vi "7 Segment LED - Automatic Counter.vi"() -> ()   [LabVIEW 2016]
panel:
  in  "STOP":bool
  out "f":bool
  out "e":bool
  out "c":bool
  out "b":bool
  out "d":bool
  out "g":bool
  out "a":bool
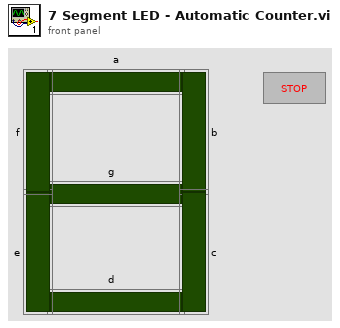
[diagram p1: front panel]
types:
  T1 = enum16{"ZERO", "ONE", "TWO", "THREE", "FOUR", "FIVE", "SIX", "SEVEN", "EIGHT", "NINE"}
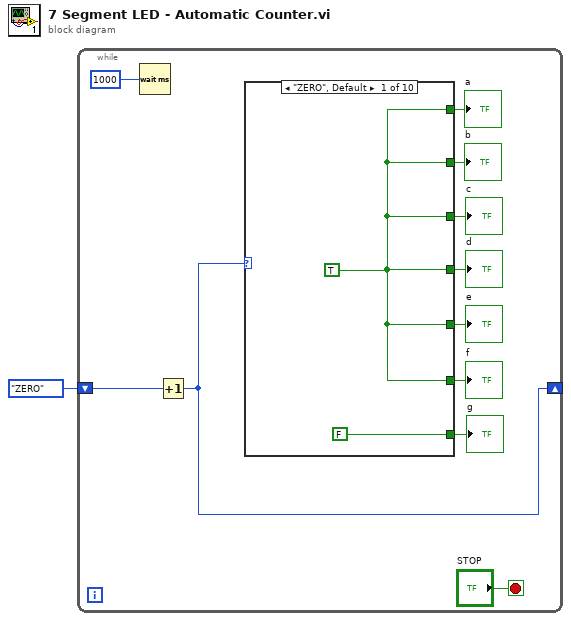
[diagram p0: block diagram]
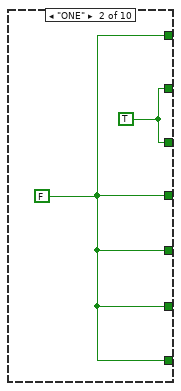
[diagram p2: hidden frame]
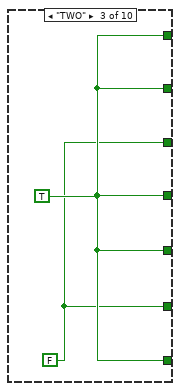
[diagram p3: hidden frame]
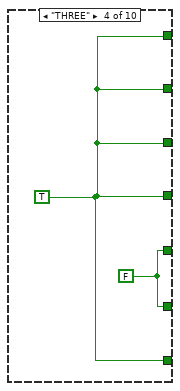
[diagram p4: hidden frame]
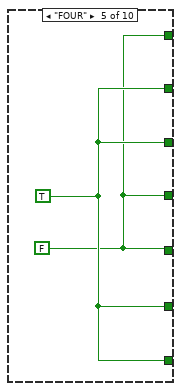
[diagram p5: hidden frame]
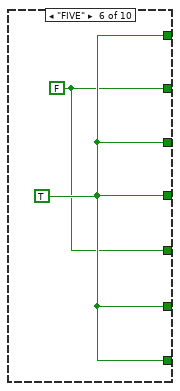
[diagram p6: hidden frame]
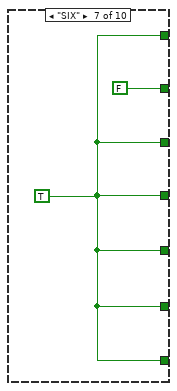
[diagram p7: hidden frame]
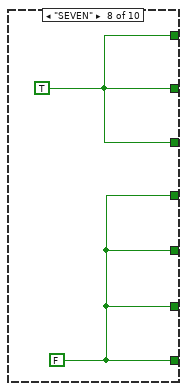
[diagram p8: hidden frame]
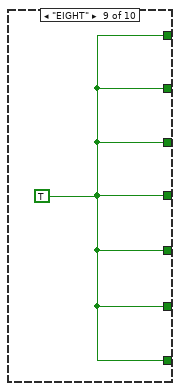
[diagram p9: hidden frame]
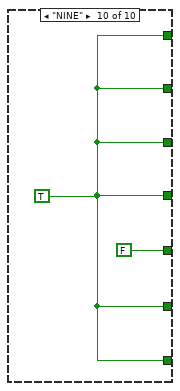
[diagram p10: hidden frame]
diagram:
  n1 = while {
    shift-right: [w2] -> _
    shift-left: T1."ZERO" ("Enum") -> [w3]
    stop <- "STOP" stop-if-true
    n2 = Wait (ms)(milliseconds to wait=1000) -> ()  [unwired: 1 out]
    n3 = Increment(x=w3) -> (x+1=w2:T1)
    n4 = case shown="\"ZERO\", Default" w2 {
      tunnel: [w14 w16 w18 w20 w21 w24 w26 w28 w29 w31] -> w10
      tunnel: [FALSE w16 w18 w20 w22 w24 w26 w27 w29 w31] -> w9
      tunnel: [w14 w16 w18 w20 w21 w24 w26 w27 w29 w31] -> w8
      tunnel: [w14 w16 w17 w19 w22 w24 w26 w27 w29 w31] -> w7
      tunnel: [w14 w16 w18 w19 w21 w23 w26 w27 w29 FALSE] -> w6
      tunnel: [w14 w15 w17 w20 w22 w24 w26 w28 w29 w31] -> w5
      tunnel: [w14 w15 w18 w20 w22 w23 FALSE w28 w29 w31] -> w4
      frame "ZERO", Default {
        w14 = TRUE
      }
      frame "ONE" {
        w15 = TRUE
        w16 = FALSE
      }
      frame "TWO" {
        w17 = FALSE
        w18 = TRUE
      }
      frame "THREE" {
        w19 = FALSE
        w20 = TRUE
      }
      frame "FOUR" {
        w21 = FALSE
        w22 = TRUE
      }
      frame "FIVE" {
        w23 = FALSE
        w24 = TRUE
      }
      frame "SIX" {
        w26 = TRUE
      }
      frame "SEVEN" {
        w27 = FALSE
        w28 = TRUE
      }
      frame "EIGHT" {
        w29 = TRUE
      }
      frame "NINE" {
        w31 = TRUE
      }
    }
    "a" <- w10
    "g" <- w9
    "d" <- w8
    "b" <- w4
    "c" <- w5
    "e" <- w6
    "f" <- w7
  }
